vi "Get measurementservice_SMULastExtCalInfoResponse.vi"(8 "error in (no error)":errorcluster, 11 "gRPCid":T3) -> (0 "error out":errorcluster, 2 "Message Data":T1, 3 "gRPCid out":T3)   [LabVIEW 2019, in "ctet_smu.lvlib" / "ctet_smu.lvclass"]
uses:
  ctet_smu.lvclass
  gRPC lvSupport/Server API/typeDefs/grpcId.ctl
  measurementservice_SMULastExtCalInfoResponse_Data.ctl
  measurementservice_ErrorOut/measurementservice_ErrorOut_Data.ctl
  a51dd2a7-b5c1-4c09-9df4-8cd9d3bd0c19.vi
  gRPC lvSupport/Server API/Server/Get Server DLL Path.vi
  gRPC lvSupport/gprc-lvsupport.lvlib
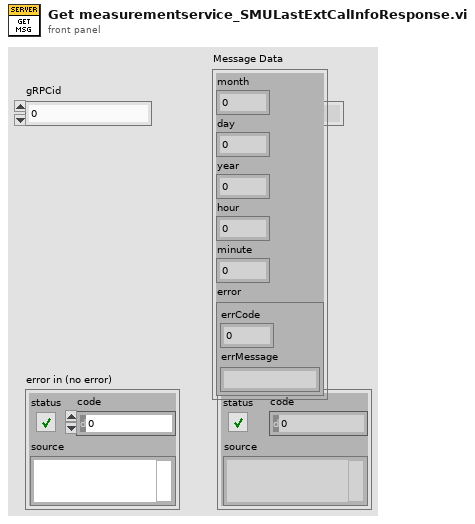
[diagram p1: front panel]
types:
  T1 = typedef "ctet_smu.lvlib/ctet_smu.lvclass/measurementservice_SMULastExtCalInfoResponse_Data.ctl" = cluster{"month":i64, "day":i64, "year":i64, "hour":i64, "minute":i64, "error":T2}
  T2 = typedef "ctet_smu.lvlib/ctet_smu.lvclass/measurementservice_ErrorOut_Data.ctl" = cluster{"errCode":i64, "errMessage":string}
  T3 = typedef "ctet_smu.lvlib/gprc-lvsupport.lvlib/grpcId.ctl" = u64
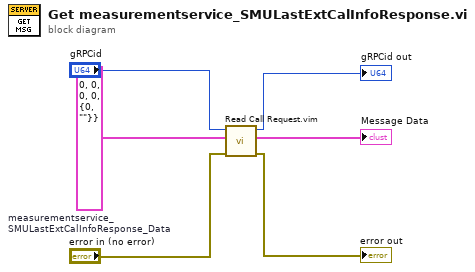
[diagram p0: block diagram]
diagram:
  w2 = T1 {"month"=0, "day"=0, "year"=0, "hour"=0, "minute"=0, "error"={"errCode"=0, "errMessage"=""}}  # measurementservice_SMULastExtCalInfoResponse_Data
  n1 = call "Read Call Request.vim"("error in (no error)"="error in (no error)", "Data Type"=w2, "gRPCid in"="gRPCid") -> ("error out"=→"error out":errorcluster, "Request Data"=→"Message Data":T1, "gRPCid out"=→"gRPCid out":T3)  [unwired: 6 in]
